vi "Sensors.vi"() -> ()   [LabVIEW 2018]
panel:
  out "IR Range":dbl
  in  "Koffset [cm]":dbl
  in  "Kscale [cm-V]":dbl=27.5
  out "Vo [V]":dbl format="%.2f"
  out "Ping Distance (m) 2":dbl
  out "Ping Distance (m) 1":dbl
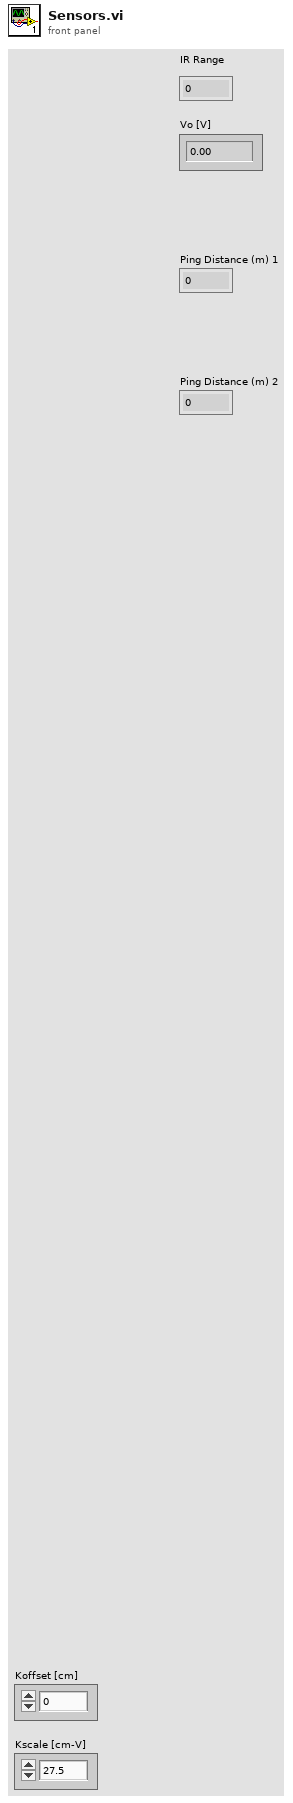
[diagram p1: front panel]
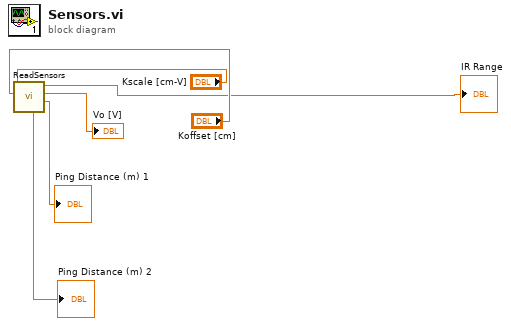
[diagram p0: block diagram]
diagram:
  n1 = call "ReadSensors.vi"("Koffset [cm]"="Koffset [cm]", "Kscale [cm-V]"="Kscale [cm-V]") -> ("Ping Distance (cm) 1"=→"Ping Distance (m) 1":dbl, "Vo [V]"=→"Vo [V]":dbl, "IR Range"=→"IR Range":dbl, "Ping Distance (cm) 2"=→"Ping Distance (m) 2":dbl)  [unwired: 6 in]
